vi "Get_Number_of_Problem_Points_in_Track_Cluster.vi"(1 "[IN] Dot Statuses":i16[][](array[numeric])) -> (0 "[OUT] Number of \npoints with problems":i32)   [LabVIEW 2013]
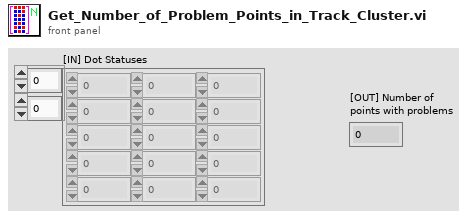
[diagram p1: front panel]
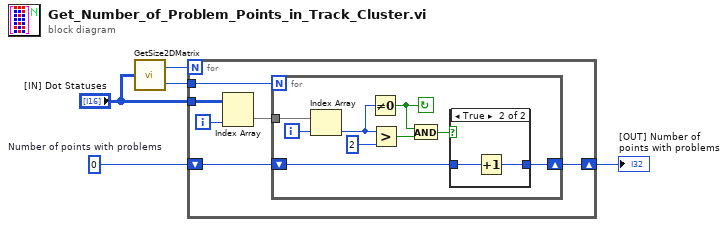
[diagram p0: block diagram]
diagram:
  w4 = 0  # Number of points with problems
  n1 = call "GetSize2DMatrix.vi"("Array IN (2D)"="[IN] Dot Statuses") -> ("# Cols"=w5:i32, "# Rows"=w2:i32)
  n2 = for {
    N: w5 -> [_]
    tunnel: w2 -> [w9]
    tunnel: "[IN] Dot Statuses" -> [w11]
    shift-right: [w6] -> w1
    shift-left: w4 -> [w7]
    i -> [w10]
    n3 = Index Array(array=w11, index (col)=w10) -> (element=w8:i16[])  [unwired: 1 in]
    n4 = for {
      N: w9 -> [_]
      tunnel: w8 -> [w20]
      shift-right: [w12] -> w6
      shift-left: w7 -> [w13]
      i -> [w19]
      stop <- w15 continue-if-true
      n5 = Index Array(array=w20, index=w19) -> (element=w18:i16)
      n6 = Not Equal To 0?(x=w18) -> (x != 0?=w15:bool)
      n7 = Greater?(x=w18, y=i16 2) -> (0:w16:bool)
      n8 = And(x=w15, y=w16) -> (x .and. y?=w14:bool)
      n9 = case shown="True" w14 {
        tunnel: w13 -> [w21 w23]
        tunnel: [w21 w22] -> w12
        frame False {
        }
        frame True {
          n10 = Increment(x=w23) -> (x+1=w22:i32)
        }
      }
    }
  }
  "[OUT] Number of \npoints with problems" <- w1
